vi "Parameters.vi"(8 "error in (no error)":errorcluster, 11 "Template Test Case In":refnum<class "Param Unit Test.lvclass">) -> (0 "error out":errorcluster, 2 "Parameters":T1(array[cluster]))   [LabVIEW 2019, in "Param Unit Test.lvclass"]
doc: "This VI defines the parameters used for execution. When LUnit runs the test case, it will run it once for every parameter in the array and collect the results.\n\nDuring test execution, the parameters are available in the class wire within the test VI."
uses:
  Param Unit Test.lvclass
  C:/Program Files (x86)/National Instruments/LabVIEW 2024/vi.lib/Astemes/LUnit Parameterized/Parameterized Test Case/Parameterized Test Case.lvclass
  <vilib>/Astemes/LUnit Parameterized/Parameterized Test Case/Parameterized Test Case.lvclass
  Parameters.ctl
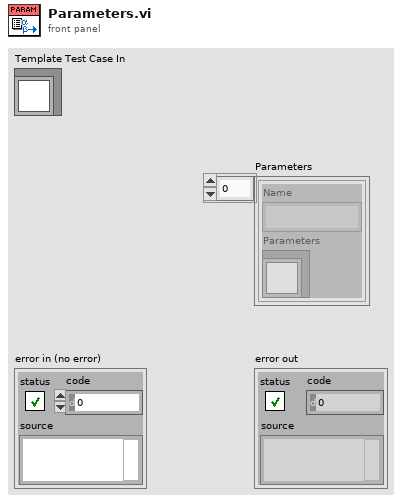
[diagram p1: front panel]
types:
  T1 = cluster{"Name":string, "Parameters":refnum<class "Parameterized Test Case.lvclass">}[]
  T2 = typedef "Param Unit Test.lvclass/Parameters.ctl" = cluster{"Command":enum16{"Set Voltage", "Set Frecuency", "Set Speed", "Set Current"}, "Input Argument":string, "Expected Command":string}
  T3 = cluster{"Scenario":string, "Parameters":refnum<class "Param Unit Test.lvclass">}[]
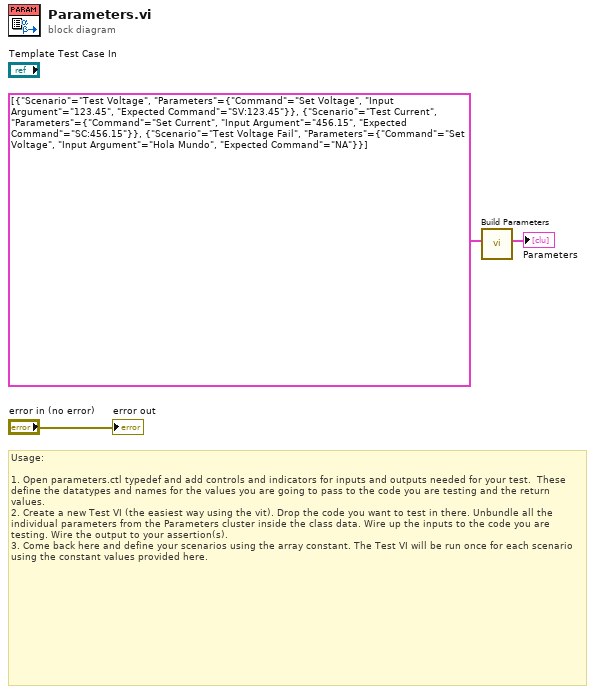
[diagram p0: block diagram]
diagram:
  # "Usage:\n\n1. Open parameters.ctl typedef and add controls and indicators for inputs and outputs needed for your test.  These define the datatypes and names for the values you are going to pass to the code you are testing and the return values.\n2. Create a new Test VI (the easiest way using the vit). Drop the code you want to test in there. Unbundle all the individual parameters from the Parameters cluster inside the class data. Wire up the inputs to the code you are testing. Wire the output to your assertion(s).\n3. Come back here and define your scenarios using the array constant. The Test VI will be run once for each scenario using the constant values provided here."
  n1 = call "Build Parameters.vi"("Scenarios In"=cluster{"Scenario":string, "Parameters":T2}[] [{"Scenario"="Test Voltage", "Parameters"={"Command"=enum."Set Voltage", "Input Argument"="123.45", "Expected Command"="SV:123.45"}}, {"Scenario"="Test Current", "Parameters"={"Command"=enum."Set Current", "Input Argument"="456.15", "Expected Command"="SC:456.15"}}, {"Scenario"="Test Voltage Fail", "Parameters"={"Command"=enum."Set Voltage", "Input Argument"="Hola Mundo", "Expected Command"="NA"}}]) -> ("Scenarios out"=→"Parameters":T3)  [unwired: 10 in]
  "error out" <- "error in (no error)"
